vi "Write Microscope Metadata.vi"(0 "File Path":path, 11 "Error In":errorcluster) -> (4 "File Path (Dup)":path, 15 "Write Errror":errorcluster)   [LabVIEW 2016]
uses:
  Microscope Modules/4Pi Capture Manager/4Pi Capture Manager Controls/4Pi Capture Notifier Type.ctl
  Microscope Modules/4Pi Capture Manager/4Pi Capture Manager Controls/4Pi Capture Actions.ctl
  Microscope Modules/4Pi Capture Manager/4Pi Capture Manager Controls/4Pi Capture Switch Line Scan Modes.ctl
  Microscope Modules/Orca Flash Capture Manager/Orca Flash Capture Manager Controls/Orca Flash Capture Notifier Type.ctl
  Microscope Modules/Orca Flash Capture Manager/Orca Flash Capture Manager Controls/Orca Flash Capture Actions.ctl
  Microscope Modules/Orca Flash Capture Manager/Orca Flash Capture Manager Controls/Orca Flash Capture Switch Line Scan Modes.ctl
  Device Metadata Types/Capture Metadata.ctl
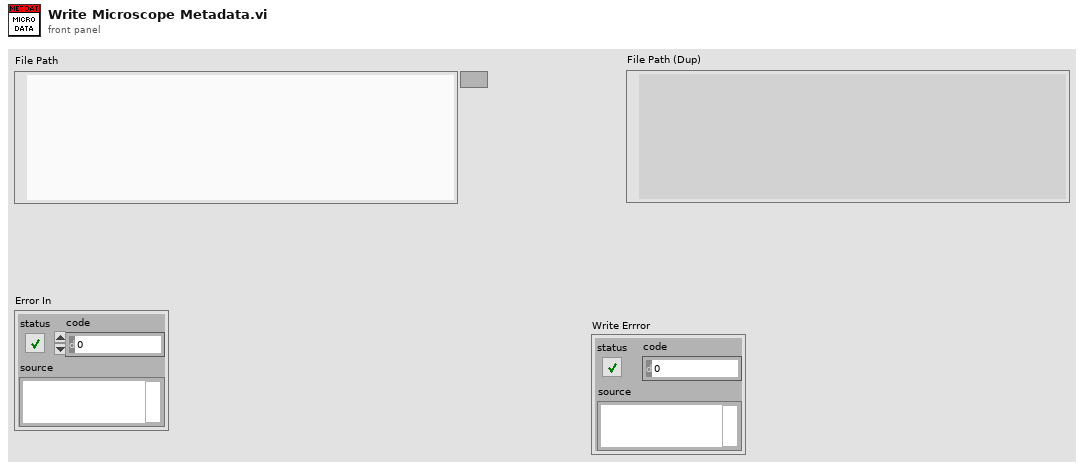
[diagram p1: front panel]
types:
  T1 = typedef "Capture Metadata.ctl" = cluster{"Capture_Exposure_sec":dbl, "Cycles":u16, "Frames":u32, "No_of_Z_Steps":u16, "Z_Step_Size_um":dbl, "Init_Z_Position_um":dbl, "Save_Path":string, "Line_Scan":bool, "Line_Scan_Mode":string}
  T2 = typedef "Orca Flash Capture Notifier Type.ctl" = cluster{"Actions":T3, "Running?":bool, "Preview Exposure (s)":dbl, "Capture Exposure (s)":dbl, "Cycles":u16, "Frames":u32, "No. of Z Steps":u16, "Z Step Size (µm)":dbl, "Base Path":path, "Init Z Position (µm)":dbl, "Save Path":path, "Line Scan?":bool, "Line Scan Mode":T4, "Collect Metadata?":bool}
  T3 = typedef "Orca Flash Capture Actions.ctl" = enum16{"Idle", "Live Preview", "Capture", "Laser On", "Laser Off", "Open Shutters", "Close Shutters", "Set Exposure Time", "Start Acquisition", "Update SubFolder", "Write Metadata", "Setup", "Camera", "Switch", "Step", "Cycle", "External Cycle Sync", "Abort", "Quit"}
  T4 = typedef "Orca Flash Capture Switch Line Scan Modes.ctl" = enum32{"Automatic", "Use Presets", "Manual"}
  T5 = typedef "4Pi Capture Notifier Type.ctl" = cluster{"Actions":T6, "Running?":bool, "Preview Exposure (s)":dbl, "Capture Exposure (s)":dbl, "Cycles":u16, "Frames":u32, "No. of Z Steps":u16, "Z Step Size (µm)":dbl, "Base Path":path, "Init Z Position (µm)":dbl, "Lasers Lines":string[], "Save Path":path, "Line Scan?":bool, "Line Scan Mode":T7, "Metadata File Ref":refnum<file>}
  T6 = typedef "4Pi Capture Actions.ctl" = enum16{"Idle", "Live Preview", "Capture", "Laser On", "Laser Off", "Open Shutters", "Close Shutters", "Set Exposure Time", "Start Acquisition", "Update SubFolder", "Setup", "Camera", "Switch", "Step", "Cycle", "External Cycle Sync", "Write Metadata", "Abort", "Quit"}
  T7 = typedef "4Pi Capture Switch Line Scan Modes.ctl" = enum32{"Automatic", "Use Presets", "Manual"}
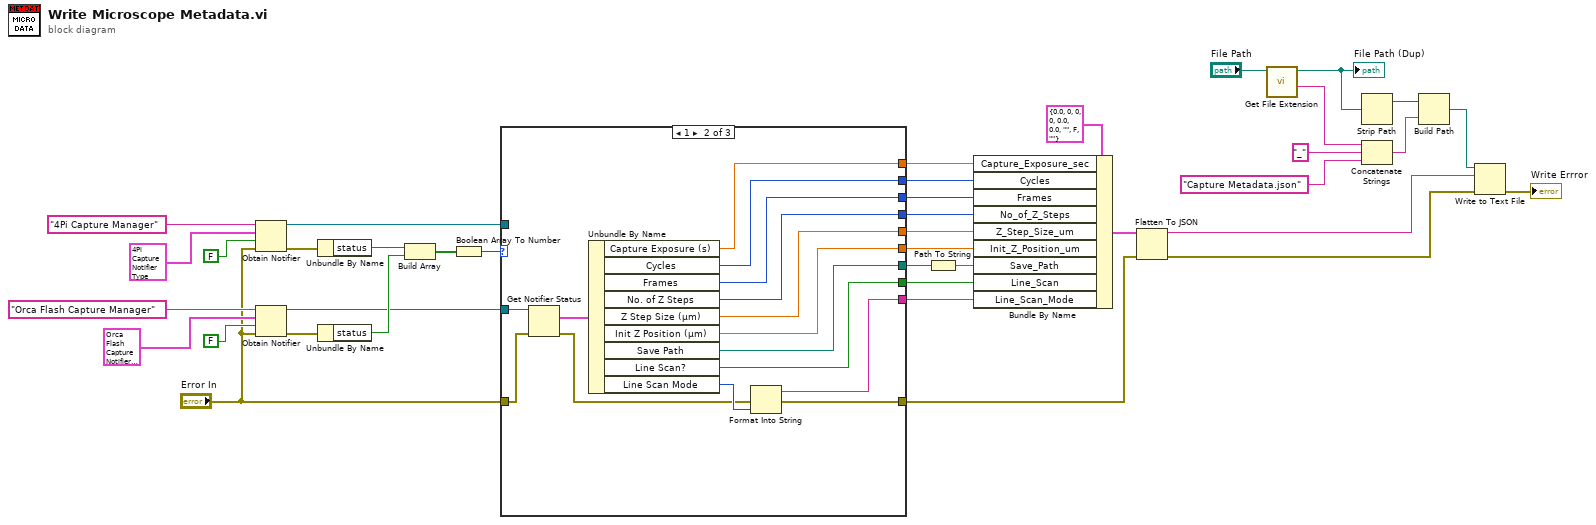
[diagram p0: block diagram]
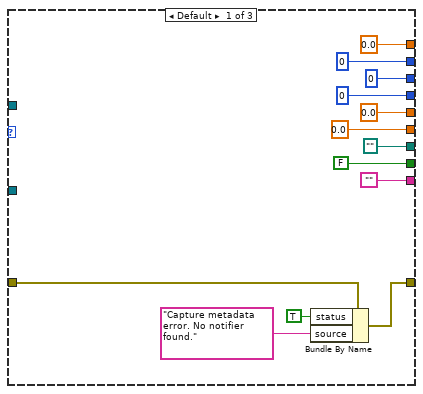
[diagram p2: hidden frame]
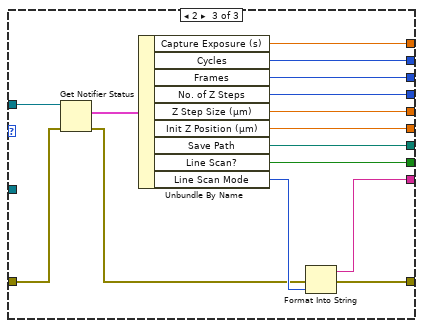
[diagram p3: hidden frame]
diagram:
  n1 = Obtain Notifier(name (unnamed)="4Pi Capture Manager", notification data type=T5 {"Actions"=enum."Live Preview", "Running?"=FALSE, "Preview Exposure (s)"=0.1, "Capture Exposure (s)"=0.1, "Cycles"=1, "Frames"=0, "No. of Z Steps"=0, "Z Step Size (µm)"=0.0, "Base Path"=path "", "Init Z Position (µm)"=0.0, "Lasers Lines"=[], "Save Path"=path "", "Line Scan?"=FALSE, "Line Scan Mode"=enum."Automatic", "Metadata File Ref"=refnum} ("4Pi Capture Notifier Type"), create if not found? (T)=FALSE, error in (no error)="Error In") -> (notifier out=w21:refnum<notifier>, error out=w27:errorcluster)  [unwired: 1 out]
  n2 = Obtain Notifier(name (unnamed)="Orca Flash Capture Manager", notification data type=T2 {"Actions"=enum."Live Preview", "Running?"=FALSE, "Preview Exposure (s)"=0.1, "Capture Exposure (s)"=0.1, "Cycles"=1, "Frames"=0, "No. of Z Steps"=0, "Z Step Size (µm)"=0.0, "Base Path"=path "", "Init Z Position (µm)"=0.0, "Save Path"=path "", "Line Scan?"=FALSE, "Line Scan Mode"=enum."Automatic", "Collect Metadata?"=FALSE} ("4Pi Capture Notifier Type"), create if not found? (T)=FALSE, error in (no error)="Error In") -> (notifier out=w20:refnum<notifier>, error out=w26:errorcluster)  [unwired: 1 out]
  n3 = Unbundle By Name(w27) -> ("status"=w25:bool)
  n4 = Unbundle By Name(w26) -> ("status"=w24:bool)
  n5 = Build Array(w25, w24) -> (w23:bool[])
  n6 = Boolean Array To Number(Boolean array=w23) -> (number=w22:u32)
  n7 = case shown="1" w22 {
    tunnel: w21 -> [_ _ w82]
    tunnel: w20 -> [_ w67 _]
    tunnel: [0.0 ("Capture Exposure (s)") w65 w80] -> w17
    tunnel: [u16 0 ("Cycles") w64 w79] -> w16
    tunnel: [u32 0 ("Frames") w63 w78] -> w15
    tunnel: [u16 0 ("No. of Z Steps") w62 w77] -> w14
    tunnel: [0.0 ("Z Step Size (µm)") w61 w76] -> w13
    tunnel: [0.0 ("Init Z Position (µm)") w60 w75] -> w12
    tunnel: [path "" w59 w74] -> w11
    tunnel: [FALSE ("Line Scan?") w58 w73] -> w9
    tunnel: ["" w56 w71] -> w8
    tunnel: "Error In" -> [w43 w54 w69]
    tunnel: [w40 w55 w70] -> w6
    frame Default {
      n8 = Bundle By Name(cluster=w43, "status"=TRUE, "source"="Capture metadata error. No notifier found.") -> (w40:errorcluster)
    }
    frame 1 {
      n9 = Get Notifier Status(notifier=w67, error in (no error)=w54) -> (current notification=w66:T2, error out=w53:errorcluster)  [unwired: 3 out]
      n10 = Unbundle By Name(w66) -> ("Capture Exposure (s)"=w65:dbl, "Cycles"=w64:u16, "Frames"=w63:u32, "No. of Z Steps"=w62:u16, "Z Step Size (µm)"=w61:dbl, "Init Z Position (µm)"=w60:dbl, "Save Path"=w59:path, "Line Scan?"=w58:bool, "Line Scan Mode"=w57:T4)
      n11 = Format Into String(error in=w53, w57) -> (resulting string=w56:string, error out=w55:errorcluster)  [unwired: 2 in]
    }
    frame 2 {
      n12 = Get Notifier Status(notifier=w82, error in (no error)=w69) -> (current notification=w81:T5, error out=w68:errorcluster)  [unwired: 3 out]
      n13 = Unbundle By Name(w81) -> ("Capture Exposure (s)"=w80:dbl, "Cycles"=w79:u16, "Frames"=w78:u32, "No. of Z Steps"=w77:u16, "Z Step Size (µm)"=w76:dbl, "Init Z Position (µm)"=w75:dbl, "Save Path"=w74:path, "Line Scan?"=w73:bool, "Line Scan Mode"=w72:T7)
      n14 = Format Into String(error in=w68, w72) -> (resulting string=w71:string, error out=w70:errorcluster)  [unwired: 2 in]
    }
  }
  n15 = Path To String(path=w11) -> (string=w10:string)
  n16 = Bundle By Name(cluster=T1 {"Capture_Exposure_sec"=0.0, "Cycles"=0, "Frames"=0, "No_of_Z_Steps"=0, "Z_Step_Size_um"=0.0, "Init_Z_Position_um"=0.0, "Save_Path"="", "Line_Scan"=FALSE, "Line_Scan_Mode"=""} ("4Pi Capture Notifier Type"), "Capture_Exposure_sec"=w17, "Cycles"=w16, "Frames"=w15, "No_of_Z_Steps"=w14, "Z_Step_Size_um"=w13, "Init_Z_Position_um"=w12, "Save_Path"=w10, "Line_Scan"=w9, "Line_Scan_Mode"=w8) -> (w18:T1)
  n17 = Flatten To JSON(anything=w18, error in (no error)=w6) -> (JSON string=w5:string, 11:w4:errorcluster)  [unwired: 1 in]
  n18 = call <vilib>:"Get File Extension.vi"("file"="File Path") -> ("filename without extension"=w1:string, "dup file"=w2:path)  [unwired: 6 in, 3 out]
  "File Path (Dup)" <- w2
  n19 = Strip Path(path=w2) -> (stripped path=w39:path)  [unwired: 1 out]
  n20 = Concatenate Strings(w1, "_" ("string"), "Capture Metadata.json" ("name or relative path")) -> (w36:string)
  n21 = Build Path(base path=w39, name or relative path=w36) -> (appended path=w35:path)
  n22 = Write to Text File(file (use dialog)=w35, text=w5, error in=w4) -> (error out=→"Write Errror":errorcluster)  [unwired: 1 in, 2 out]
